vi "WriteSF_basic.vi"(7 "Connection ID":refnum<k5>, 8 "MsgType":u8, 9 "Destination ID":u16, 11 "Servo Positions":T1={"Data0"=100, "Data1"=100, "Data2"=100, "Data3"=100, "Data4"=100, "Data5"=100, "Data6"=100, "Data7"=100}) -> ()   [LabVIEW 2011]
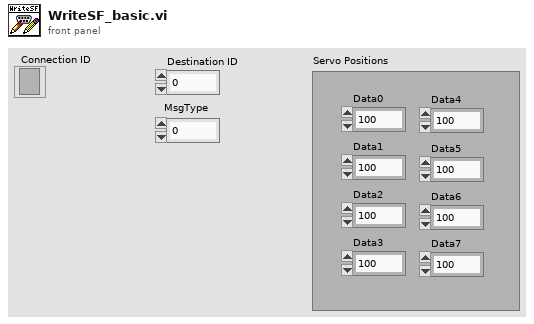
[diagram p1: front panel]
types:
  T1 = cluster{"Data0":u8, "Data1":u8, "Data2":u8, "Data3":u8, "Data4":u8, "Data5":u8, "Data6":u8, "Data7":u8}
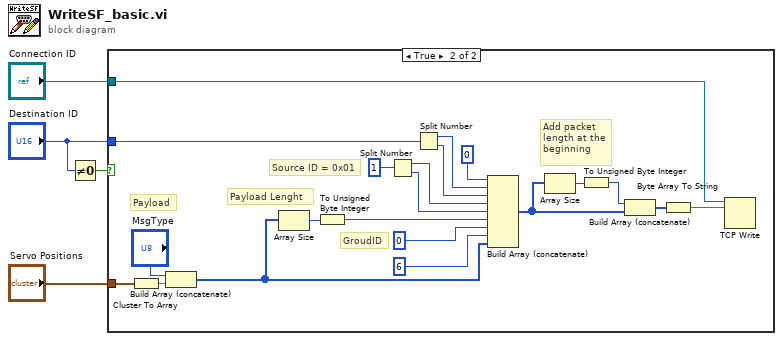
[diagram p0: block diagram]
diagram:
  n1 = Not Equal To 0?(x="Destination ID") -> (x != 0?=w4:bool)
  n2 = case shown="True" w4 {
    tunnel: "Destination ID" -> [_ w8]
    tunnel: "Connection ID" -> [_ w7]
    tunnel: "Servo Positions" -> [_ w5]
    frame False {
    }
    frame True {
      # "Add packet\nlength at the\nbeginning"
      # "Payload"
      # "GroudID"
      # "Payload Lenght"
      # "Source ID = 0x01"
      n3 = Cluster To Array(cluster=w5) -> (array=w6:u8[])
      n4 = Build Array (concatenate)("MsgType", w6) -> (w19:u8[])
      n5 = Array Size(array=w19) -> (size(s)=w18:i32)
      n6 = To Unsigned Byte Integer(number=w18) -> (unsigned 8bit integer=w17:u8)
      n7 = Split Number(x=u16 1 ("Actuator ID\nBlue")) -> (hi(x)=w11:u8, lo(x)=w10:u8)
      n8 = Split Number(x=w8) -> (hi(x)=w22:u8, lo(x)=w21:u8)
      n9 = Build Array (concatenate)(u8 0, w22, w21, w11, w10, w17, u8 0, u8 6, w19) -> (w15:u8[])
      n10 = Array Size(array=w15) -> (size(s)=w14:i32)
      n11 = To Unsigned Byte Integer(number=w14) -> (unsigned 8bit integer=w13:u8)
      n12 = Build Array (concatenate)(w13, w15) -> (w12:u8[])
      n13 = Byte Array To String(unsigned byte array=w12) -> (string=w16:string)
      n14 = TCP Write(connection ID=w7, data in=w16) -> ()  [unwired: 2 in, 3 out]
    }
  }
